vi "Create Object.vi"(11 "Dev Panel in":refnum<class "Dev Panel.lvclass">) -> (3 "Dev Panel out":refnum<class "Dev Panel.lvclass">)   [LabVIEW 2021, in "Dev Panel.lvclass"]
uses:
  Dev Panel.lvclass
  Dev Panel.lvclass/Dev Panel.ctl
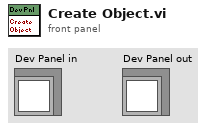
[diagram p1: front panel]
types:
  T1 = cluster{"Events":cluster{"Teardown":refnum<user-event>, "Pop Up":refnum<user-event>, "String Indicator":refnum<user-event>, "Button":refnum<user-event>}, "Refs":cluster{"Pop Up":refnum<vi>, "String Indicator":refnum<vi>, "Button":refnum<vi>}, "BG Color":u32}
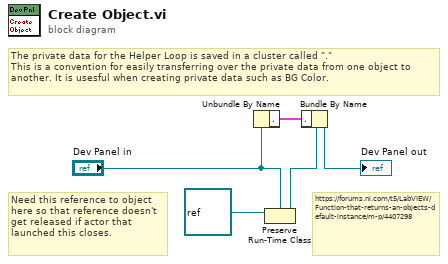
[diagram p0: block diagram]
diagram:
  # "The private data for the Helper Loop is saved in a cluster called \".\"\nThis is a convention for easily transferring over the private data from one object to another. It is usesful when creating private data such as BG Color."
  # "https://forums.ni.com/t5/LabVIEW/Function-that-returns-an-objects-default-instance/m-p/4407298"
  # "Need this reference to object here so that reference doesn't get released if actor that launched this closes."
  n1 = Unbundle By Name("Dev Panel in") -> ("."=w5:T1)
  n2 = Preserve Run-Time Class(object in=refnum<class> refnum ("LabVIEW Object"), 2:"Dev Panel in") -> (object out=w3:refnum<class "Dev Panel.lvclass">)  [unwired: 1 in, 1 out]
  n3 = Bundle By Name(cluster=w3, "."=w5) -> (→"Dev Panel out":refnum<class "Dev Panel.lvclass">)
